vi "Valves State.vi"(8 "error in (no error)":errorcluster, 11 "Syringe in":refnum<class "Syringe Line.lvclass">) -> (0 "error out":errorcluster, 1 "Valve Capillar Open":bool, 2 "Valve Transfer Line Open":bool, 3 "Syringe out":refnum<class "Syringe Line.lvclass">)   [LabVIEW 2015, in "cRIO-Carbondioxide.lvlib" / "CO2-Actor.lvlib" / "Syringe Line.lvclass"]
uses:
  Syringe Line.lvclass
  Valve/Valve.lvclass
  Syringe Line.lvclass/Syringe Line.ctl
  CO2 Actor Messages/Ping Msg/Ping Msg.lvclass/Ping Msg.ctl
  <vilib>/ActorFramework/Message Enqueuer/Message Enqueuer.lvclass/Message Enqueuer.ctl
  <vilib>/ActorFramework/Message Enqueuer/Enqueue.vi
  <vilib>/ActorFramework/Message Priority Queue/Priority Enqueue.vi
  CO2 Actor Messages/Ping Msg/Ping Msg.lvclass
  <vilib>/ActorFramework/Actor/Actor.lvclass
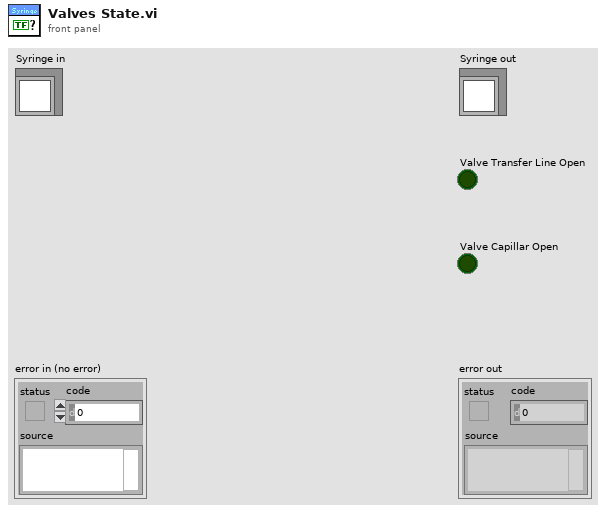
[diagram p1: front panel]
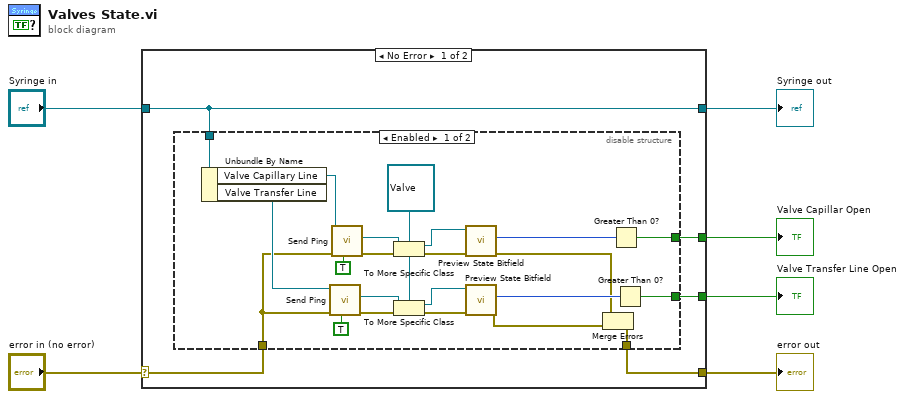
[diagram p0: block diagram]
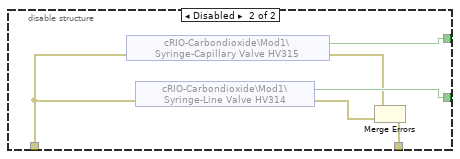
[diagram p2: hidden frame]
diagram:
  n1 = case shown="No Error" "error in (no error)" {
    selector: "error in (no error)" -> [w7 w41]
    tunnel: [w11 w41] -> w5
    tunnel: [w8 w40] -> w3
    tunnel: "Syringe in" -> [w8 w40]
    tunnel: [w10 _] -> w2
    tunnel: [w9 _] -> w1
    frame No Error {
      n2 = disable-structure shown="Enabled" {
        disable-tunnel: [w24 w39] -> w11
        disable-tunnel: [w19 w34] -> w10
        disable-tunnel: [w18 w36] -> w9
        disable-tunnel: w8 -> [w16 _]
        disable-tunnel: w7 -> [w15 w38]
        frame Enabled {
          w29 = refnum<class "Valve.lvclass"> refnum ("Valve.lvclass")
          n3 = Unbundle By Name(w16) -> ("Valve Capillary Line"=w14:refnum<class "Message Enqueuer.lvclass">, "Valve Transfer Line"=w17:refnum<class "Message Enqueuer.lvclass">)
          n4 = call "Send Ping.vi"("Return Self (F)"=TRUE, "error in (no error)"=w15, "Message Enqueuer"=w17) -> ("error out"=w30:errorcluster, "Actor out"=w22:refnum<class "Actor.lvclass">)  [unwired: 5 in, 2 out]
          n5 = call "Send Ping.vi"("Return Self (F)"=TRUE, "error in (no error)"=w15, "Message Enqueuer"=w14) -> ("error out"=w31:errorcluster, "Actor out"=w23:refnum<class "Actor.lvclass">)  [unwired: 5 in, 2 out]
          n6 = To More Specific Class(target class=w29, reference=w23, error in=w31) -> (specific class reference=w27:refnum<class "Valve.lvclass">, error out=w28:errorcluster)
          n7 = To More Specific Class(target class=w29, reference=w22, error in=w30) -> (specific class reference=w25:refnum<class "Valve.lvclass">, error out=w26:errorcluster)
          n8 = call "Preview State Bitfield.vi"("error in (no error)"=w28, "Valve in"=w27) -> ("error out"=w13:errorcluster, "State Bitfield"=w21:u16)  [unwired: 7 in, 1 out]
          n9 = call "Preview State Bitfield.vi"("error in (no error)"=w26, "Valve in"=w25) -> ("error out"=w12:errorcluster, "State Bitfield"=w20:u16)  [unwired: 7 in, 1 out]
          n10 = Merge Errors(w13, w12) -> (w24:errorcluster)
          n11 = Greater Than 0?(x=w21) -> (x > 0?=w19:bool)
          n12 = Greater Than 0?(x=w20) -> (x > 0?=w18:bool)
        }
        frame Disabled {
          n13 = shared-variable "cRIO-Carbondioxide\\Mod1\\Syringe-Capillary Valve HV315"(error in=w38) -> (w34:bool, error out=w35:errorcluster)
          n14 = shared-variable "cRIO-Carbondioxide\\Mod1\\Syringe-Line Valve HV314"(error in=w38) -> (w36:bool, error out=w37:errorcluster)
          n15 = Merge Errors(w35, w37) -> (w39:errorcluster)
        }
      }
    }
    frame Error {
    }
  }
  "error out" <- w5
  "Syringe out" <- w3
  "Valve Capillar Open" <- w2
  "Valve Transfer Line Open" <- w1
